vi "niSwitch DMM-array.vi"() -> ()   [LabVIEW 2017]
doc: "I. Description:\n\nThis example demonstrates how to scan a series of channels on a switch module and take measurements with an NI digital multimeter using handshaking. \n\nHANDSHAKING:\nFirst, the DMM is initiated and waits for a digital pulse from the switch before taking any measurements. When the switch scanning task is started, it connects the first channel in its scan list, waits for the channel to settle and generates a digital pulse-Scan Advanced. When the DMM receives this digital pulse, it takes the first measurement and generates a digital pulse-Measurement Complete (MC). When the switch receives this digital pulse, it advances to the next entry in its scan list and this continues.\n\nII. Instructions for Running:\n\nTo make this example work with your switch, complete the following:\nSWITCH SETUP: (refer to the NI Switches Help) \nEnter the DAQmx/traditional DAQ switch resource name.\nSelect the correct topology for your switch module.\nEnter a valid scan list.\nSelect valid values for Trigger Input and Scan Advanced Output. \n\nDMM SETUP: (refer to your NI DMM documentation)\nEnter the DAQmx/traditional DAQ DMM resource name.\nSelect measurement type, range and resolution.\nEnter number of samples.\nSelect a valid Measurement Complete Destination and Trigger Source.\n\nRefer to the NI Switches Help to determine if your switch supports scanning, the scan list syntax, and the valid channel names and valid resource names for your switch module.\n\nIII. Block Diagram Steps:\n\nA) The switch is configured first. Triggers and scan list are set. The scanning configuration is downloaded to the hardware with niSwitch Commit.vi.\nB) The DMM is configured. Functions, range, resolution, triggers and number of points to take are set. When the DMM initiates, it configures its hardware according to the settings and waits for a trigger. \nC) When the switch initiates it connects the first channels in its scan list, waits for the relays to settle and send its Scan Advanced signal to trigger the DMM for its first measurement. Once the DMM has taken a measurement, the DMM sends its MC signal to the switch to advance to the next entry in the scan list. \nD) The DMM returns to the user the number of measurements specified in \"Samples to Fetch at a Time\". When the stop button is pushed the acquisition stops.\nE) Terminates the scanning operation, closes the session to the switch, and displays errors if any.\n\nIV. I/O Connections Overview:\n\nRefer to the NI Switches Getting Started Guide and NI Switches Help for information about connecting signals to your switch module."
uses:
  <instrlib>/niDMM/nidmm.llb/niDMM Function.ctl
  <instrlib>/niDMM/nidmm.llb/niDMM Trigger.ctl
  <instrlib>/niSwitch/niSwitch.llb/niSwitch Topologies.ctl
  <instrlib>/niDMM/nidmm.llb/niDMM Sample Trigger.ctl
  <instrlib>/niDMM/nidmm.llb/niDMM Configure Measurement Absolute.vi
  <vilib>/Utility/NIReport.llb/Append Text Table to Report (wrap).vi
  <vilib>/Utility/NIReport.llb/NI_report.lvclass
panel:
  out "转置的数组":dbl[][](array[numeric])=[[5.8333333333243935, 6.666666666658539, 10.83333333332927, 3.3333333333219555, 1.666666666668292, 0.0, 2.500000000002438, 13.333333333331707], [9.166666666660978, 1.666666666668292, 10.83333333332927, 1.666666666668292, 9.166666666660978, 8.333333333326832, 5.8333333333243935, 8.333333333326832], [1.666666666668292, 5.8333333333243935, 9.166666666660978, 4.999999999990248, 7.499999999992686, 14.166666666665854, 4.166666666656102, 4.999999999990248], [12.499999999997563, 2.500000000002438, 12.499999999997563, 14.166666666665854, 9.166666666660978, 0.0, 4.166666666656102, 4.166666666656102], [14.166666666665854, 13.333333333331707, 15.0, 12.499999999997563, 14.166666666665854, 5.8333333333243935, 0.0, 5.8333333333243935], [1.666666666668292, 14.166666666665854, 14.166666666665854, 0.0, 8.333333333326832, 5.8333333333243935, 4.999999999990248, 15.0], [0.0, 14.166666666665854, 15.0, 9.166666666660978, 13.333333333331707, 2.500000000002438, 8.333333333326832, 1.666666666668292], [11.666666666663415, 7.499999999992686, 2.500000000002438, 0.0, 12.499999999997563, 7.499999999992686, 2.500000000002438, 8.333333333326832]]
  in  "选项卡控件":enum32{"强度图", "数据"}(tab)=enum."数据"
  out "强度图":dbl[][](graph)=[[5.8333333333243935, 6.666666666658539, 10.83333333332927, 3.3333333333219555, 1.666666666668292, 0.0, 2.500000000002438, 13.333333333331707], [9.166666666660978, 1.666666666668292, 10.83333333332927, 1.666666666668292, 9.166666666660978, 8.333333333326832, 5.8333333333243935, 8.333333333326832], [1.666666666668292, 5.8333333333243935, 9.166666666660978, 4.999999999990248, 7.499999999992686, 14.166666666665854, 4.166666666656102, 4.999999999990248], [12.499999999997563, 2.500000000002438, 12.499999999997563, 14.166666666665854, 9.166666666660978, 0.0, 4.166666666656102, 4.166666666656102], [14.166666666665854, 13.333333333331707, 15.0, 12.499999999997563, 14.166666666665854, 5.8333333333243935, 0.0, 5.8333333333243935], [1.666666666668292, 14.166666666665854, 14.166666666665854, 0.0, 8.333333333326832, 5.8333333333243935, 4.999999999990248, 15.0], [0.0, 14.166666666665854, 15.0, 9.166666666660978, 13.333333333331707, 2.500000000002438, 8.333333333326832, 1.666666666668292], [11.666666666663415, 7.499999999992686, 2.500000000002438, 0.0, 12.499999999997563, 7.499999999992686, 2.500000000002438, 8.333333333326832]]
  out "Measurements":dbl[](array[numeric])=[0.5000221359436212, 0.5000031622776602, 0.4999905131670195, 0.4999873508893593, 0.49999367544467965, 0.5000284604989416, 0.49997786405637884, 0.5000031622776602, 0.499981026334039, 0.49999367544467965, 0.4999873508893593, 0.4999873508893593, 0.4999715395010585, 0.4999905131670195, 0.5000031622776602, 0.499981026334039, 0.4999715395010585, 0.5000031622776602, 0.5000252982212814, 0.4999715395010585, 0.49999367544467965, 0.49999367544467965, 0.499981026334039, 0.5, 0.49997786405637884, 0.5000063245553203, 0.5, 0.5000063245553203, 0.5000252982212814, 0.5000031622776602, 0.5000221359436212, 0.500018973665961, 0.49998418861169913, 0.49997786405637884, 0.4999905131670195, 0.5000252982212814, 0.500018973665961, 0.4999715395010585, 0.5000063245553203, 0.4999715395010585, 0.5000126491106407, 0.5000126491106407, 0.5000063245553203, 0.500018973665961, 0.5000284604989416, 0.5000252982212814, 0.5000284604989416, 0.499981026334039, 0.4999968377223398, 0.49997786405637884, 0.49999367544467965, 0.499981026334039, 0.5000221359436212, 0.5000252982212814, 0.5000252982212814, 0.5, 0.49999367544467965, 0.5000063245553203, 0.49997786405637884, 0.500018973665961, 0.5000252982212814, 0.49997786405637884, 0.4999715395010585, 0.5000158113883009] caption="原始数据" format="%.7f"
  out "归一化数据":dbl[](array[numeric])=[13.333333333331707, 8.333333333326832, 4.999999999990248, 4.166666666656102, 5.8333333333243935, 15.0, 1.666666666668292, 8.333333333326832, 2.500000000002438, 5.8333333333243935, 4.166666666656102, 4.166666666656102, 0.0, 4.999999999990248, 8.333333333326832, 2.500000000002438, 0.0, 8.333333333326832, 14.166666666665854, 0.0, 5.8333333333243935, 5.8333333333243935, 2.500000000002438, 7.499999999992686, 1.666666666668292, 9.166666666660978, 7.499999999992686, 9.166666666660978, 14.166666666665854, 8.333333333326832, 13.333333333331707, 12.499999999997563, 3.3333333333219555, 1.666666666668292, 4.999999999990248, 14.166666666665854, 12.499999999997563, 0.0, 9.166666666660978, 0.0, 10.83333333332927, 10.83333333332927, 9.166666666660978, 12.499999999997563, 15.0, 14.166666666665854, 15.0, 2.500000000002438, 6.666666666658539, 1.666666666668292, 5.8333333333243935, 2.500000000002438, 13.333333333331707, 14.166666666665854, 14.166666666665854, 7.499999999992686, 5.8333333333243935, 9.166666666660978, 1.666666666668292, 12.499999999997563, 14.166666666665854, 1.666666666668292, 0.0, 11.666666666663415]
  out "输出数组":dbl[][](array[numeric])=[[13.333333333331707, 8.333333333326832, 4.999999999990248, 4.166666666656102, 5.8333333333243935, 15.0, 1.666666666668292, 8.333333333326832], [2.500000000002438, 5.8333333333243935, 4.166666666656102, 4.166666666656102, 0.0, 4.999999999990248, 8.333333333326832, 2.500000000002438], [0.0, 8.333333333326832, 14.166666666665854, 0.0, 5.8333333333243935, 5.8333333333243935, 2.500000000002438, 7.499999999992686], [1.666666666668292, 9.166666666660978, 7.499999999992686, 9.166666666660978, 14.166666666665854, 8.333333333326832, 13.333333333331707, 12.499999999997563], [3.3333333333219555, 1.666666666668292, 4.999999999990248, 14.166666666665854, 12.499999999997563, 0.0, 9.166666666660978, 0.0], [10.83333333332927, 10.83333333332927, 9.166666666660978, 12.499999999997563, 15.0, 14.166666666665854, 15.0, 2.500000000002438], [6.666666666658539, 1.666666666668292, 5.8333333333243935, 2.500000000002438, 13.333333333331707, 14.166666666665854, 14.166666666665854, 7.499999999992686], [5.8333333333243935, 9.166666666660978, 1.666666666668292, 12.499999999997563, 14.166666666665854, 1.666666666668292, 0.0, 11.666666666663415]]
  in  "error in (no error)":errorcluster caption="错误输入（无错误）"
  in  "Save":bool caption="Stop"
  out "大小":i32=64
  in  "通道个数":i32=64 min=9 max=64
  in  "Maximum Time (msec)":i32=5000
  in  "topology name":T1="2530/2-Wire 64x1 Mux"
  in  "measurement type":T2=enum."DC Current"
  in  "trigger source":T3=enum."TTL 7"
  in  "range":dbl=0.5 format="%.2f"
  in  "resolution":dbl=1e-05 format="%.0p"
  in  "scan advanced output":T4(ring)=enum."TTL7"
  in  "trigger input":T5(ring)=enum."TTL0"
  in  "measurement complete destination":u16(ring)=2 items=["None", "External", "TTL 0", "TTL 1", "TTL 2", "TTL 3", "TTL 4", "TTL 5", "TTL 6", "TTL 7", "LBR Trig 0"]
  in  "resource name":refnum<k15>="PXI1Slot5"
  out "scan list":string="ch0:63->com0;"
  in  "resource name":refnum<k15>="PXI1Slot6"
  in  "Stop":bool
  # "SWITCH"
  # "DMM"
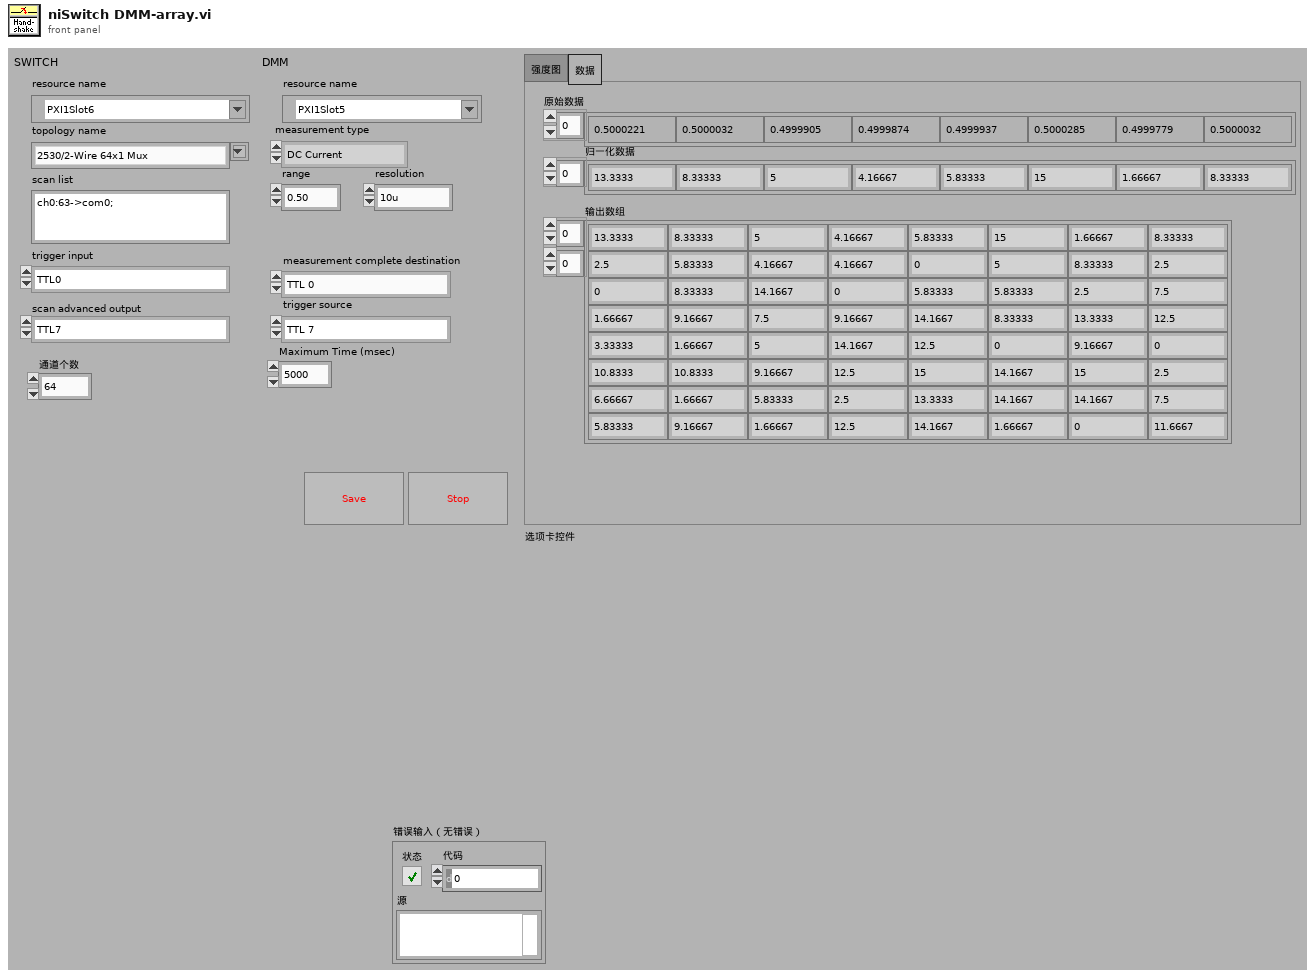
[diagram p1: front panel]
types:
  T1 = typedef "niSwitch Topologies.ctl" = string
  T2 = typedef "niDMM Function.ctl" = enum16{"DC Volts", "AC Volts", "DC Current", "AC Current", "2-wire Resistance", "4-wire Resistance", "Diode", "Frequency", "Period", "AC Volts DC Coupled", "Capacitance", "Inductance", "Temperature"}
  T3 = typedef "niDMM Trigger.ctl" = enum16{"Immediate", "External", "TTL 0", "TTL 1", "TTL 2", "TTL 3", "TTL 4", "TTL 5", "TTL 6", "Software", "TTL 7", "PXI Star", "LBR Trig 1", "Aux Trig 1"}
  T4 = enum16{"None", "External", "TTL0", "TTL1", "TTL2", "TTL3", "TTL4", "TTL5", "TTL6", "TTL7", "ECL0", "ECL1", "PXI Star", "Rear Connector", "Front Connector", "Rear Connector Module 1", "Rear Connector Module 2", "Rear Connector Module 3", "Rear Connector Module 4", "Rear Connector Module 5", "Rear Connector Module 6", "Rear Connector Module 7", "Rear Connector Module 8", "Rear Connector Module 9", "Rear Connector Module 10", "Rear Connector Module 11", "Rear Connector Module 12", "Front Connector Module 1", "Front Connector Module 2", "Front Connector Module 3", "Front Connector Module 4", "Front Connector Module 5", "Front Connector Module 6", "Front Connector Module 7", "Front Connector Module 8", "Front Connector Module 9", "Front Connector Module 10", "Front Connector Module 11", "Front Connector Module 12"}
  T5 = enum16{"Immediate", "External", "TTL0", "TTL1", "TTL2", "TTL3", "TTL4", "TTL5", "TTL6", "TTL7", "ECL0", "ECL1", "PXI Star", "Software Trigger Function", "Rear Connector", "Front Connector", "Rear Connector of Module 1", "Rear Connector of Module 2", "Rear Connector of Module 3", "Rear Connector of Module 4", "Rear Connector of Module 5", "Rear Connector of Module 6", "Rear Connector of Module 7", "Rear Connector of Module 8", "Rear Connector of Module 9", "Rear Connector of Module 10", "Rear Connector of Module 11", "Rear Connector of Module 12", "Front Connector of Module 1", "Front Connector of Module 2", "Front Connector of Module 3", "Front Connector of Module 4", "Front Connector of Module 5", "Front Connector of Module 6", "Front Connector of Module 7", "Front Connector of Module 8", "Front Connector of Module 9", "Front Connector of Module 10", "Front Connector of Module 11", "Front Connector of Module 12"}
  T6 = typedef "niDMM Sample Trigger.ctl" = enum16{"Immediate", "External", "TTL 0", "TTL 1", "TTL 2", "TTL 3", "TTL 4", "TTL 5", "TTL 6", "Interval", "Software", "TTL 7", "PXI Star", "LBR Trig 1", "Aux Trig 1"}
  T7 = enum16{"maximized", "minimized", "normal", "no change"}
  T8 = enum16{"Standard Report", "HTML", "Word", "Excel"}
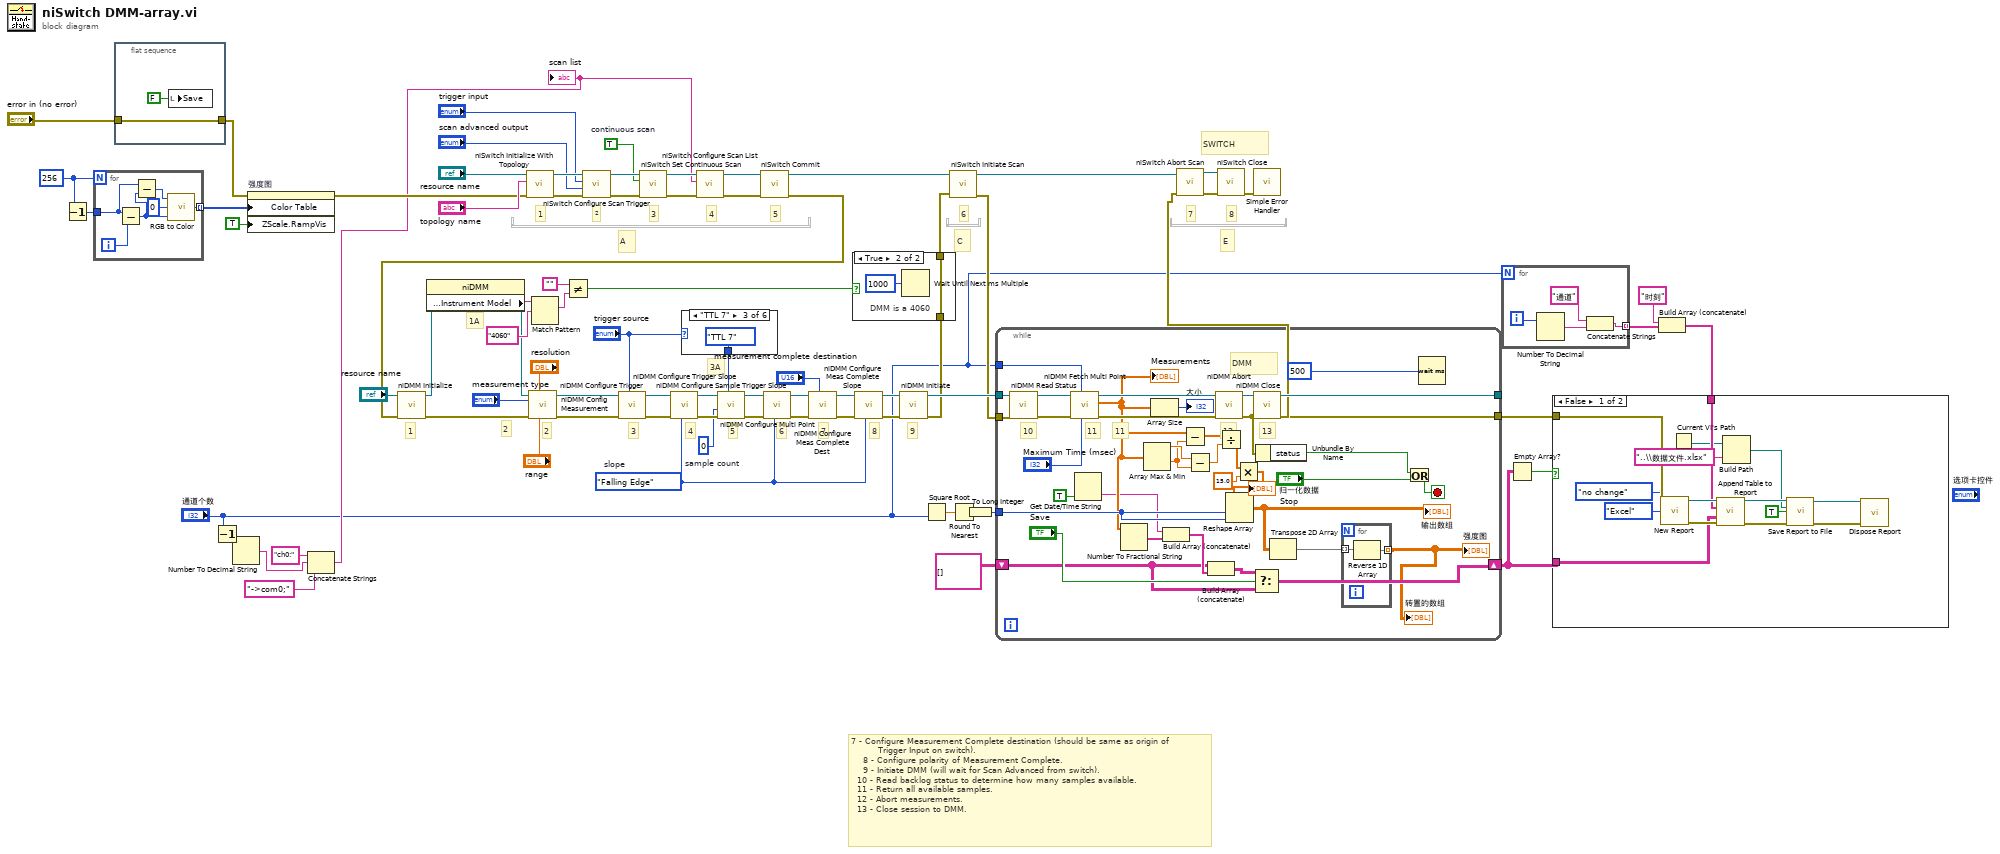
[diagram p0: block diagram]
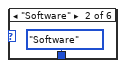
[diagram p5: hidden frame]
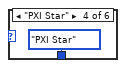
[diagram p6: hidden frame]
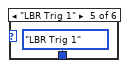
[diagram p7: hidden frame]
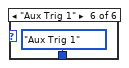
[diagram p8: hidden frame]
diagram:
  w21 = 256
  w43 = enum16{"Rising Edge", "Falling Edge"}."Falling Edge"  # slope
  w59 = 0  # sample count
  w77 = TRUE  # continuous scan
  # "2"
  # "5"
  # "7 - Configure Measurement Complete destination (should be same as origin of\n         Trigger Input on switch).\n    8 - Configure polarity of Measurement Complete.\n    9 - Initiate DMM (will wait for Scan Advanced from switch).\n  10 - Read backlog status to determine how many samples available.  \n  11 - Return all available samples.\n  12 - Abort measurements.\n  13 - Close session to DMM."
  # "9"
  # "13"
  # "12"
  # "8"
  # "3A"
  # "1A"
  # "4"
  # "6"
  # "11"
  # "5"
  # "7"
  # "3"
  # "2"
  # "1"
  # "E"
  # "C"
  # "A"
  # "DMM"
  # "SWITCH"
  # "6"
  # "8"
  # "7"
  # "4"
  # "3"
  # "2"
  # "1"
  n1 = Decrement(x=w21) -> (x-1=w20:i32)
  n2 = for {
    N: w21 -> [_]
    tunnel: w20 -> [w86]
    tunnel: [w82] -> w19 mode=indexing
    i -> [w87]
    n3 = Subtract(x=w86, y=w87) -> (x-y=w85:i32)
    n4 = Subtract(x=w86, y=w85) -> (x-y=w84:i32)
    n5 = call <vilib>:"RGB to Color.vi"("B"=w85, "G"=u8 0, "R"=w84) -> ("Color"=w82:u32)
  }
  n6 = flat-sequence {
    tunnel: "error in (no error)" -> [w88]
    tunnel: [w88] -> w3
    frame #0 {
      n7 = local write "Save"(FALSE ("Save")) -> ()
    }
  }
  n8 = Decrement(x="通道个数") -> (x-1=w13:i32)
  n9 = Number To Decimal String(number=w13) -> (decimal integer string=w16:string)  [unwired: 1 in]
  n10 = property on="强度图" class="IntGraph (strict)"(error in=w3, "Color Table"=w19, "ZScale.RampVis"=TRUE ("Z标尺.颜色梯度可见")) -> (error out=w18:errorcluster)  [unwired: 1 in, 1 out]
  n11 = Concatenate Strings("ch0:" ("字符串"), w16, "->com0;" ("字符串")) -> (w14:string)
  "scan list" <- w14
  n12 = call <instrlib>:"niSwitch Initialize With Topology.vi"("error in (no error)"=w18, "topology name"="topology name", "resource name"="resource name") -> ("error out"=w73:errorcluster, "instrument handle out"=w74:refnum<k15>)  [unwired: 7 in]
  n13 = call <instrlib>:"niSwitch Configure Scan Trigger.vi"("error in (no error)"=w73, "scan advanced output (External)"="scan advanced output", "trigger input (External)"="trigger input", "instrument handle"=w74) -> ("error out"=w78:errorcluster, "instrument handle out"=w80:refnum<k15>)  [unwired: 6 in]
  n14 = call <instrlib>:"niSwitch Set Continuous Scan.vi"("error in (no error)"=w78, "continuous scan (False)"=w77, "instrument handle"=w80) -> ("error out"=w71:errorcluster, "instrument handle out"=w72:refnum<k15>)  [unwired: 7 in]
  n15 = case shown="\"TTL 7\"" "trigger source" {
    selector: "trigger source" -> [w90 _ _ _ _ _]
    tunnel: [w90 niDMM_Sample_Trigger."Software" ("Sample Trigger") niDMM_Sample_Trigger."TTL 7" ("Sample Trigger") niDMM_Sample_Trigger."PXI Star" ("Sample Trigger") niDMM_Sample_Trigger."LBR Trig 1" ("Sample Trigger") niDMM_Sample_Trigger."Aux Trig 1" ("Sample Trigger")] -> w57
    frame "Immediate", Default {
    }
    frame "Software" {
    }
    frame "TTL 7" {
    }
    frame "PXI Star" {
    }
    frame "LBR Trig 1" {
    }
    frame "Aux Trig 1" {
    }
  }
  n16 = call <instrlib>:"niSwitch Configure Scan List.vi"("error in (no error)"=w71, "scan list"=w14, "instrument handle"=w72) -> ("error out"=w37:errorcluster, "instrument handle out"=w36:refnum<k15>)  [unwired: 7 in]
  n17 = call <instrlib>:"niSwitch Commit.vi"("error in (no error)"=w37, "instrument handle"=w36) -> ("error out"=w35:errorcluster, "instrument handle out"=w34:refnum<k15>)  [unwired: 8 in]
  n18 = call <instrlib>:"niDMM Initialize.vi"("error in (no error)"=w35, "Instrument Descriptor"="resource name") -> ("error out"=w29:errorcluster, "instrument handle out"=w39:refnum<k15>)  [unwired: 8 in]
  n19 = property class="niDMM"(reference=w39) -> (reference out=w32:refnum<k15>, "Inherent IVI Attributes:Instrument Identification:Instrument Model"=w40:string)  [unwired: 1 in, 1 out]
  n20 = call-poly <instrlib>:"niDMM Config Measurement.vi"("Range"="range", "Resolution"="resolution", "error in (no error)"=w29, "Function"="measurement type", "instrument handle"=w32) -> ("error out"=w26:errorcluster, "instrument handle out"=w27:refnum<k15>)  [unwired: 5 in]
  n21 = Match Pattern(string=w40, regular expression="4060") -> (match substring=w54:string)  [unwired: 1 in, 3 out]
  n22 = Not Equal?(x="", y=w54) -> (x != y?=w52:bool)
  n23 = call <instrlib>:"niDMM Configure Trigger.vi"("Trigger Source"="trigger source", "error in (no error)"=w26, "instrument handle"=w27) -> ("error out"=w64:errorcluster, "instrument handle out"=w65:refnum<k15>)  [unwired: 7 in]
  n24 = call <instrlib>:"niDMM Configure Trigger Slope.vi"("Slope"=w43, "error in (no error)"=w64, "instrument handle"=w65) -> ("error out"=w62:errorcluster, "instrument handle out"=w63:refnum<k15>)  [unwired: 7 in]
  n25 = call <instrlib>:"niDMM Configure Multi Point.vi"("Sample Trigger"=w57, "error in (no error)"=w62, "Sample Count"=w59, "instrument handle"=w63) -> ("error out"=w60:errorcluster, "instrument handle out"=w61:refnum<k15>)  [unwired: 6 in]
  n26 = call <instrlib>:"niDMM Configure Sample Trigger Slope.vi"("Slope"=w43, "error in (no error)"=w60, "instrument handle"=w61) -> ("error out"=w50:errorcluster, "instrument handle out"=w49:refnum<k15>)  [unwired: 7 in]
  n27 = call <instrlib>:"niDMM Configure Meas Complete Dest.vi"("Measurement Complete Destination"="measurement complete destination", "error in (no error)"=w50, "instrument handle"=w49) -> ("error out"=w44:errorcluster, "instrument handle out"=w47:refnum<k15>)  [unwired: 7 in]
  n28 = call <instrlib>:"niDMM Configure Meas Complete Slope.vi"("Slope"=w43, "error in (no error)"=w44, "instrument handle"=w47) -> ("error out"=w45:errorcluster, "instrument handle out"=w46:refnum<k15>)  [unwired: 7 in]
  n29 = call <instrlib>:"niDMM Initiate.vi"("error in (no error)"=w45, "instrument handle"=w46) -> ("error out"=w56:errorcluster, "instrument handle out"=w69:refnum<k15>)  [unwired: 8 in]
  n30 = case shown="True" w52 {
    tunnel: w56 -> [w96 w97]
    tunnel: [w96 w97] -> w51
    frame False {
      # "DMM is \nnot a 4060"
    }
    frame True {
      # "DMM is a 4060"
      n31 = Wait Until Next ms Multiple(millisecond multiple=u32 1000) -> ()  [unwired: 1 out]
    }
  }
  n32 = Square Root(x="通道个数") -> (sqrt(x)=w24:dbl)
  n33 = call <instrlib>:"niSwitch Initiate Scan.vi"("error in (no error)"=w51, "instrument handle"=w34) -> ("error out"=w11:errorcluster, "instrument handle out"=w70:refnum<k15>)  [unwired: 8 in]
  n34 = Round To Nearest(number=w24) -> (nearest integer value=w23:dbl)
  n35 = To Long Integer(number=w23) -> (32bit integer=w22:i32)
  n36 = while {
    tunnel: [w131] -> w58
    tunnel: w69 -> [w127]
    tunnel: [w130] -> w9
    tunnel: w11 -> [w124]
    tunnel: w22 -> [w121]
    tunnel: "通道个数" -> [w118]
    shift-right: [w103] -> w2
    shift-left: string[][] [] -> [w104]
    stop <- w122 stop-if-true
    # "11"
    # "10"
    # "9"
    n37 = call <instrlib>:"niDMM Read Status.vi"("error in (no error)"=w124, "instrument handle"=w127) -> ("error out"=w126:errorcluster, "instrument handle out"=w125:refnum<k15>)  [unwired: 6 in, 2 out]
    n38 = call <instrlib>:"niDMM Fetch Multi Point.vi"("Maximum Time (msec)"="Maximum Time (msec)", "Number to Fetch"=w118, "error in (no error)"=w126, "instrument handle"=w125) -> ("error out"=w130:errorcluster, "Measurements"=w109:dbl[], "instrument handle out"=w131:refnum<k15>)  [unwired: 4 in, 1 out]
    "Measurements" <- w109
    n39 = Get Date/Time String(want seconds? (F)=TRUE ("需要秒？(F)")) -> (time string=w108:string)  [unwired: 2 in, 1 out]
    n40 = Number To Fractional String(number=w109) -> (F-format string=w107:string[])  [unwired: 3 in]
    n41 = Array Max & Min(array=w109) -> (max value=w117:dbl, min value=w116:dbl)  [unwired: 2 out]
    n42 = Array Size(array=w109) -> (size(s)=→"大小":i32)
    n43 = Build Array (concatenate)(w108, w107) -> (w106:string[])
    n44 = Subtract(x=w109, y=w116) -> (x-y=w115:dbl[])
    n45 = Subtract(x=w117, y=w116) -> (x-y=w114:dbl)
    n46 = Build Array (concatenate)(w104, w106) -> (w105:string[][])
    n47 = Divide(x=w115, y=w114) -> (x/y=w113:dbl[])
    n48 = Multiply(x=w113, y=15.0) -> (x*y=w111:dbl[])
    "归一化数据" <- w111
    n49 = Reshape Array(w111, w121, w121) -> (w101:dbl[][])
    "输出数组" <- w101
    n50 = Select(t=w105, s="Save", f=w104) -> (s? t:f=w103:string[][])
    n51 = Unbundle By Name(w130) -> ("status"=w129:bool)
    n52 = Transpose 2D Array(2D array=w101) -> (transposed array=w100:dbl[][])
    n53 = for {
      tunnel: w100 -> [w133] mode=indexing
      tunnel: [w132] -> w99 mode=indexing
      n54 = Reverse 1D Array(array=w133) -> (reversed array=w132:dbl[])
    }
    "强度图" <- w99
    "转置的数组" <- w99
    n55 = Or(x=w129, y="Stop") -> (x .or. y?=w122:bool)
    n56 = Wait (ms)(milliseconds to wait=u32 500 ("等待时间（毫秒）")) -> ()  [unwired: 1 out]
  }
  n57 = call <instrlib>:"niDMM Abort.vi"("error in (no error)"=w9, "instrument handle"=w58) -> ("error out"=w67:errorcluster, "instrument handle out"=w68:refnum<k15>)  [unwired: 8 in]
  n58 = call <instrlib>:"niDMM Close.vi"("error in (no error)"=w67, "instrument handle"=w68) -> ("error out"=w38:errorcluster)  [unwired: 9 in]
  n59 = call <instrlib>:"niSwitch Abort Scan.vi"("error in (no error)"=w38, "instrument handle"=w70) -> ("error out"=w76:errorcluster, "instrument handle out"=w79:refnum<k15>)  [unwired: 8 in]
  n60 = call <instrlib>:"niSwitch Close.vi"("error in (no error)"=w76, "instrument handle"=w79) -> ("error out"=w81:errorcluster)  [unwired: 9 in]
  n61 = call <vilib>:"Simple Error Handler.vi"("error in (no error)"=w81) -> ()  [unwired: 4 in, 5 out]
  n62 = for {
    N: "通道个数" -> [_]
    tunnel: [w134] -> w6 mode=indexing
    i -> [w137]
    n63 = Number To Decimal String(number=w137) -> (decimal integer string=w136:string)  [unwired: 1 in]
    n64 = Concatenate Strings("通道" ("字符串"), w136) -> (w134:string)
  }
  n65 = Empty Array?(array=w2) -> (empty?=w1:bool)
  n66 = Build Array (concatenate)("时刻", w6) -> (w5:string[])
  n67 = case shown="False" w1 {
    tunnel: w9 -> [w151 _]
    tunnel: w5 -> [w148 _]
    tunnel: w2 -> [w138 _]
    frame False {
      n68 = call <vilib>:"New Report.vi"("window state (normal)"=T7."no change", "report type"=T8."Excel", "error in (no error)"=w151) -> ("report out"=w150:refnum<class "NI_report.lvclass">, "error out"=w149:errorcluster)  [unwired: 11 in]
      n69 = Current VI's Path() -> (path=w144:path)
      n70 = call-poly <vilib>:"Append Table to Report.vi"("report in"=w150, "column headers"=w148, "text data"=w138, "error in (no error)"=w149) -> ("report out"=w147:refnum<class "NI_report.lvclass">, "error out"=w146:errorcluster)  [unwired: 8 in, 2 out]
      n71 = Build Path(base path=w144, name or relative path="..\\数据文件.xlsx" ("名称或相对路径")) -> (appended path=w142:path)
      n72 = call-dynamic "Save Report to File.vi"("report in"=w147, "report file path"=w142, "prompt to replace? (F)"=TRUE, "error in (no error)"=w146) -> ("report out"=w140:refnum<class "NI_report.lvclass">, "error out"=w141:errorcluster)  [unwired: 10 in]
      n73 = call-dynamic "Dispose Report.vi"("report in"=w140, "error in (no error)"=w141) -> ()  [unwired: 13 in, 1 out]
    }
    frame True {
    }
  }
